vi "Discovery Client Unregister Service.vi"(5 "Request Data":T2, 11 "error in (no error)":errorcluster) -> (6 "Response Data":T1, 15 "error out":errorcluster)   [LabVIEW 2020]
uses:
  Discovery Client_lv/Discovery_client/RPC Messages/ni_measurementlink_discovery_v1_UnregisterServiceRequest.ctl
  Discovery Client_lv/Discovery_client/RPC Messages/ni_measurementlink_discovery_v1_UnregisterServiceResponse.ctl
  Discovery Client_lv/Discovery_client/Discovery_client.lvlib
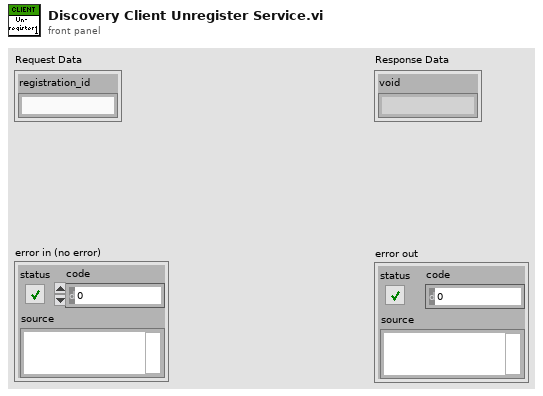
[diagram p1: front panel]
types:
  T1 = typedef "Discovery_client.lvlib/ni_measurementlink_discovery_v1_UnregisterServiceResponse.ctl" = cluster{"void":string}
  T2 = typedef "Discovery_client.lvlib/ni_measurementlink_discovery_v1_UnregisterServiceRequest.ctl" = cluster{"registration_id":string}
  T3 = typedef "grpc-lvsupport-release.lvlib/grpcId.ctl" = u64
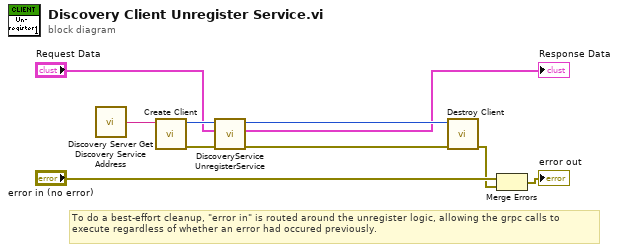
[diagram p0: block diagram]
diagram:
  # "To do a best-effort cleanup, \"error in\" is routed around the unregister logic, allowing the grpc calls to execute regardless of whether an error had occured previously."
  n1 = call "Discovery Server Get Discovery Service Address.vi"() -> ("address"=w10:string)  [unwired: 15 in]
  n2 = call "Create Client.vi"("address"=w10) -> ("error out"=w9:errorcluster, "gRPC ID Out"=w8:T3)  [unwired: 9 in]
  n3 = call "DiscoveryService UnregisterService.vi"("error in"=w9, "Request Data"="Request Data", "gRPC ID"=w8) -> ("error out"=w7:errorcluster, "Response Data"=→"Response Data":T1, "gRPC ID out"=w6:T3)  [unwired: 6 in]
  n4 = call "Destroy Client.vi"("error in"=w7, "gRPC ID"=w6) -> ("error out"=w2:errorcluster)  [unwired: 9 in]
  n5 = Merge Errors("error in (no error)", w2) -> (→"error out":errorcluster)
